vi "test.DataChangeFilter.vi"() -> ()   [LabVIEW 2017]
uses:
  7d50e549-d73b-4641-aba5-3dd9bdc8a104.vi
panel:
  in  "Reset(F)":bool
  out "Array 3":dbl[](array[numeric])
  out "check data 2":dbl[](array[numeric])
  in  "Array 2":dbl[](array[numeric])
  in  "check data":dbl[](array[numeric])
  in  "stop":bool
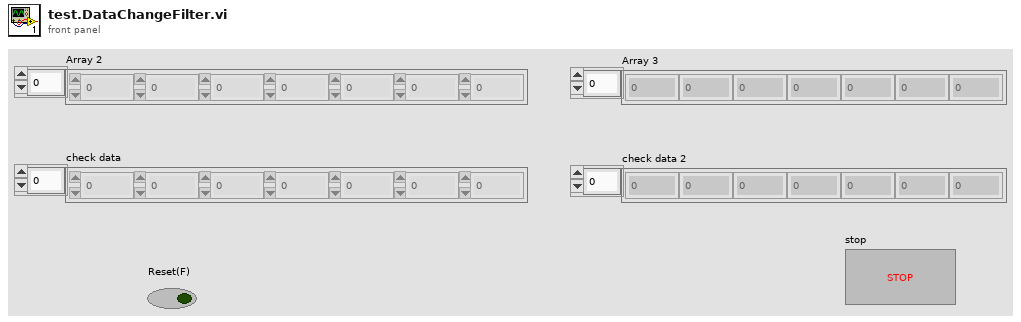
[diagram p1: front panel]
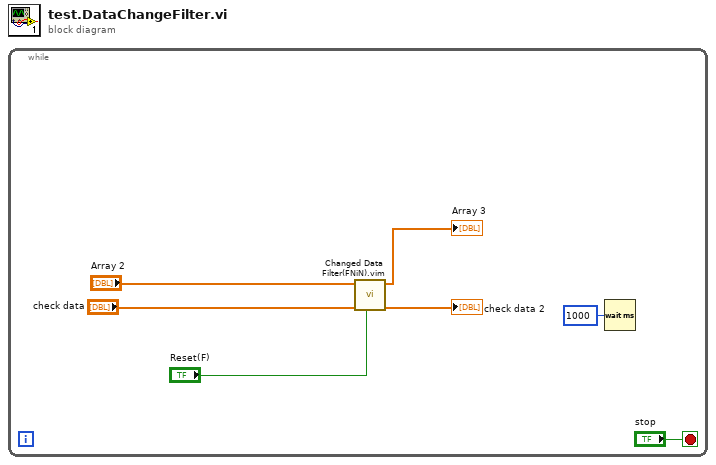
[diagram p0: block diagram]
diagram:
  n1 = while {
    stop <- "stop" stop-if-true
    n2 = call "Changed Data Filter(FNiN).vim"("Reset(F)"="Reset(F)", "checked data"="check data", "1"="Array 2") -> ("data"=→"check data 2":dbl[], "1 out"=→"Array 3":dbl[])  [unwired: 5 in, 2 out]
    n3 = Wait (ms)(milliseconds to wait=u32 1000) -> ()  [unwired: 1 out]
  }
